vi "Asylum_GetDate.vi"(8 "error in (no error)":errorcluster, 11 "Application":refnum<k7>) -> (0 "error out":errorcluster, 2 "results":string, 3 "Application":refnum<k7>)   [LabVIEW 2016]
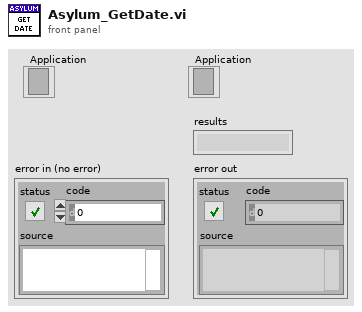
[diagram p1: front panel]
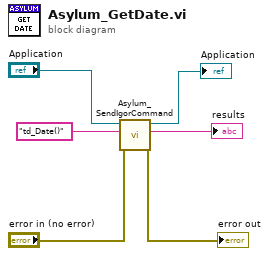
[diagram p0: block diagram]
diagram:
  n1 = call "Asylum_SendIgorCommand.vi"("error in (no error)"="error in (no error)", "command"="td_Date()", "Application"="Application") -> ("error out"=→"error out":errorcluster, "results"=→"results":string, "Application"=→"Application":refnum<k7>)  [unwired: 5 in, 1 out]
